vi "lineProfileCalculator.vi"(6 "ZoomInteger":cluster{"X":i32, "Y":i32}, 7 "Image":T1(plugin-control), 8 "error in (no error)":errorcluster, 9 "Displayed Image Size":cluster{"Width":u32, "Height":u32}, 10 "Image Center Position":cluster{"X":u32, "Y":u32}, 11 "Snapper in":refnum<class "Snapper.lvclass">) -> (0 "error out":errorcluster, 1 "y profile":cluster{"Pixels Line":sgl[], i32[]}(graph), 2 "X Profile":cluster{"x0":sgl, "dx":sgl, "Pixels Line":sgl[]}(graph), 3 "Snapper out":refnum<class "Snapper.lvclass">, 4 "Image out":T1(plugin-control))   [LabVIEW 2011, in "Views.lvlib" / "Camera.lvlib" / "Snapper.lvclass"]
uses:
  Snapper.lvclass
  <vilib>/vision/NI_Vision_Development_Module.lvlib
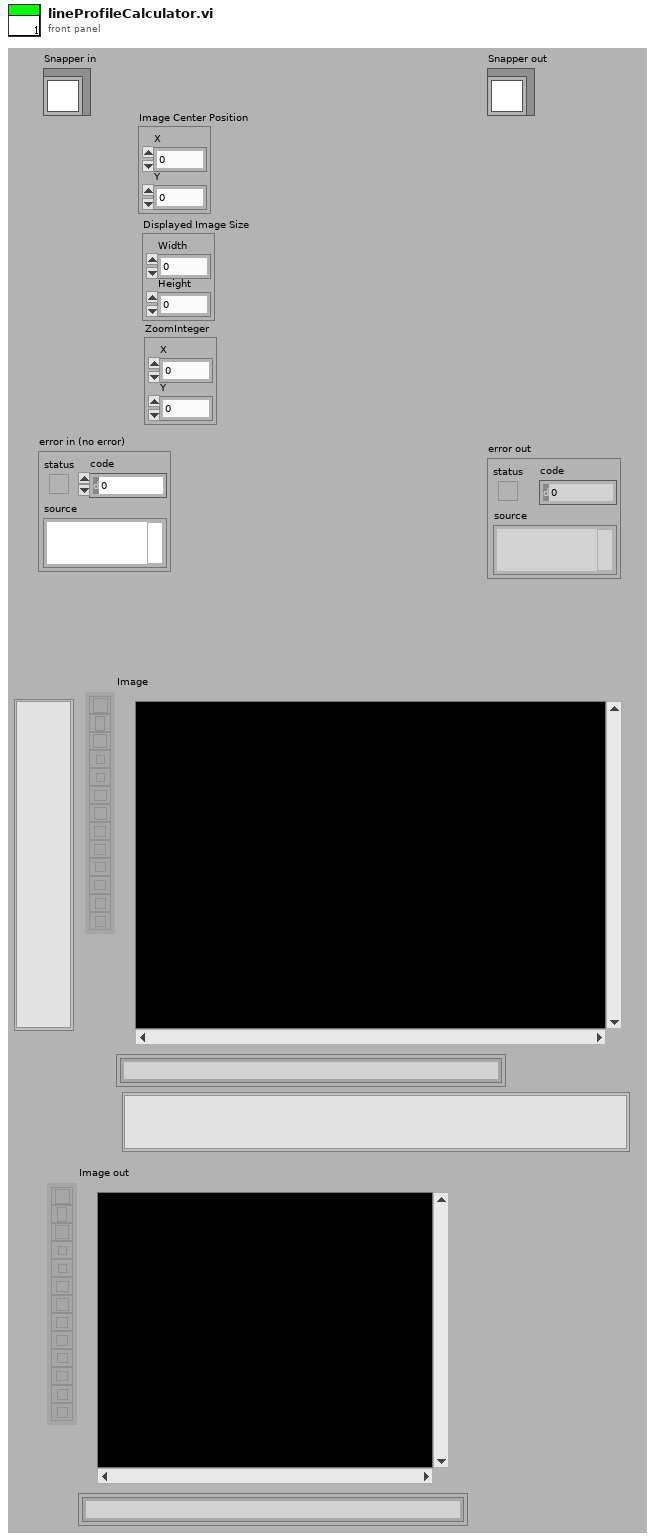
[diagram p1: front panel]
types:
  T1 = typedef "IMAQ Image.ctl" = refnum<image>
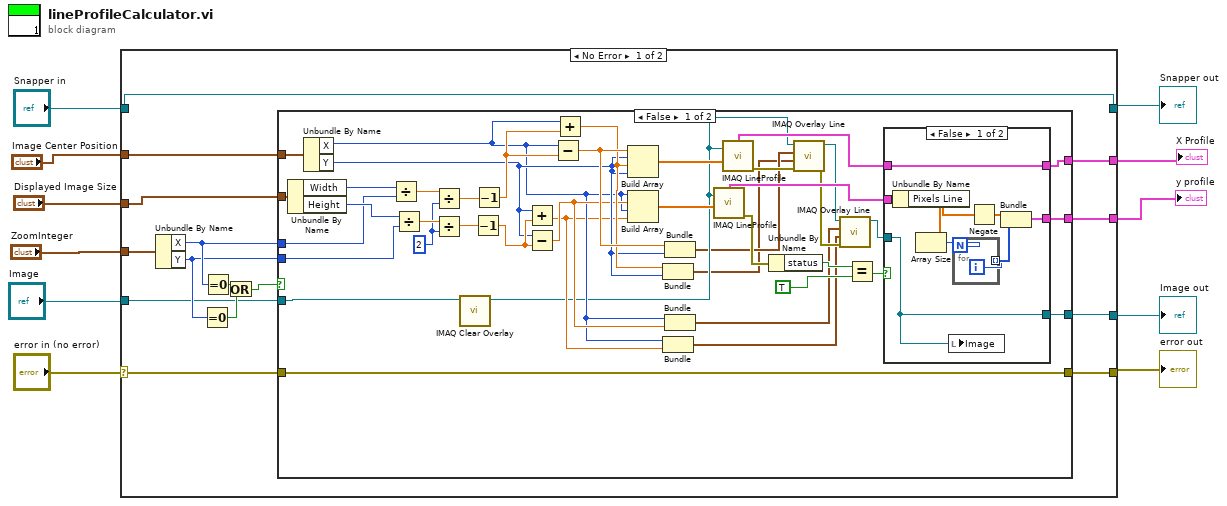
[diagram p0: block diagram]
diagram:
  n1 = case shown="No Error" "error in (no error)" {
    selector: "error in (no error)" -> [w22 w82]
    tunnel: [w21 w82] -> w10
    tunnel: [w26 w81] -> w8
    tunnel: "Snapper in" -> [w26 w81]
    tunnel: "Image Center Position" -> [w25 _]
    tunnel: "Displayed Image Size" -> [w24 _]
    tunnel: "ZoomInteger" -> [w23 _]
    tunnel: "Image" -> [w14 w80]
    tunnel: [w20 _] -> w3
    tunnel: [w19 _] -> w2
    tunnel: [w12 w80] -> w1
    frame No Error {
      n2 = Unbundle By Name(w23) -> ("X"=w18:i32, "Y"=w17:i32)
      n3 = Equal To 0?(x=w17) -> (x = 0?=w15:bool)
      n4 = Equal To 0?(x=w18) -> (x = 0?=w16:bool)
      n5 = Or(x=w16, y=w15) -> (x .or. y?=w13:bool)
      n6 = case shown="False" w13 {
        tunnel: w25 -> [w58 _]
        tunnel: w24 -> [w57 _]
        tunnel: w22 -> [w50 w79]
        tunnel: w14 -> [w27 w78]
        tunnel: [w50 w79] -> w21
        tunnel: [w45 _] -> w20
        tunnel: [w53 _] -> w19
        tunnel: w18 -> [w52 _]
        tunnel: w17 -> [w51 _]
        tunnel: [w28 w78] -> w12
        frame False {
          w65 = 2
          n7 = Unbundle By Name(w57) -> ("Width"=w64:u32, "Height"=w63:u32)
          n8 = Unbundle By Name(w58) -> ("X"=w36:u32, "Y"=w38:u32)
          n9 = Divide(x=w64, y=w52) -> (x/y=w67:dbl)
          n10 = Divide(x=w63, y=w51) -> (x/y=w66:dbl)
          n11 = Divide(x=w67, y=w65) -> (x/y=w61:dbl)
          n12 = Divide(x=w66, y=w65) -> (x/y=w62:dbl)
          n13 = call "IMAQ Clear Overlay"("Image"=w27) -> ("Image Out"=w33:T1)  [unwired: 9 in, 1 out]
          n14 = Decrement(x=w62) -> (x-1=w59:dbl)
          n15 = Decrement(x=w61) -> (x-1=w60:dbl)
          n16 = Add(x=w38, y=w59) -> (x+y=w35:dbl)
          n17 = Subtract(x=w38, y=w59) -> (x-y=w37:dbl)
          n18 = Subtract(x=w36, y=w60) -> (x-y=w40:dbl)
          n19 = Add(x=w36, y=w60) -> (x+y=w39:dbl)
          n20 = Build Array(w40, w38, w39, w38) -> (w56:dbl[])
          n21 = Build Array(w36, w37, w36, w35) -> (w55:dbl[])
          n22 = Bundle(w39, "Y"=w38) -> (w31:cluster{dbl, "Y":u32})  [unwired: 1 in]
          n23 = Bundle("X"=w36, w35) -> (w30:cluster{"X":u32, dbl})  [unwired: 1 in]
          n24 = Bundle(w40, "Y"=w38) -> (w32:cluster{dbl, "Y":u32})  [unwired: 1 in]
          n25 = Bundle("X"=w36, w37) -> (w29:cluster{"X":u32, dbl})  [unwired: 1 in]
          n26 = call "IMAQ LineProfile"("Line Coordinates"=w55, "Image"=w33) -> ("error out"=w43:errorcluster, "Line Graph"=w54:cluster{"x0":sgl, "dx":sgl, "Pixels Line":sgl[]})  [unwired: 3 in, 2 out]
          n27 = call "IMAQ LineProfile"("Line Coordinates"=w56, "Image"=w33) -> ("error out"=w44:errorcluster, "Line Graph"=w46:cluster{"x0":sgl, "dx":sgl, "Pixels Line":sgl[]})  [unwired: 3 in, 2 out]
          n28 = Unbundle By Name(w43) -> ("status"=w49:bool)
          n29 = call "IMAQ Overlay Line"("error in (no error)"=w44, "End Point"=w31, "Start Point"=w32, "Image"=w33) -> ("error out"=w42:errorcluster, "Image Out"=w41:T1)  [unwired: 6 in]
          n30 = call "IMAQ Overlay Line"("error in (no error)"=w42, "End Point"=w30, "Start Point"=w29, "Image"=w41) -> ("Image Out"=w34:T1)  [unwired: 6 in, 1 out]
          n31 = Equal?(x=w49, y=TRUE) -> (x = y?=w47:bool)
          n32 = case shown="False" w47 {
            tunnel: w54 -> [w71 _]
            tunnel: [w70 _] -> w53
            tunnel: w46 -> [w69 _]
            tunnel: [w69 _] -> w45
            tunnel: w34 -> [w68 w77]
            tunnel: [w68 w77] -> w28
            frame False {
              n33 = Unbundle By Name(w71) -> ("Pixels Line"=w72:sgl[])
              n34 = Array Size(array=w72) -> (size(s)=w74:i32)
              n35 = local write "Image"(w68) -> ()
              n36 = for {
                N: w74 -> [_]
                tunnel: [w76] -> w73 mode=indexing
                i -> [w76]
              }
              n37 = Negate(x=w72) -> (-x=w75:sgl[])
              n38 = Bundle(w75, w73) -> (w70:cluster{sgl[], i32[]})  [unwired: 1 in]
            }
            frame True {
            }
          }
        }
        frame True {
        }
      }
    }
    frame Error {
    }
  }
  "error out" <- w10
  "Snapper out" <- w8
  "X Profile" <- w3
  "y profile" <- w2
  "Image out" <- w1
